vi "Manager Launcher.vi"() -> ()   [LabVIEW 2021, in "CIF Engine Launch.lvlib"]
uses:
  CIF Engine Launch.lvlib
  CIFUtilities/CIFLogs/Typedef/Message Type.ctl
  CIFUtilities/CIFConfigurationFile/typedef/Location Type.ctl
  363d3bde-6874-4068-849e-62e045d4c070.vi
  CIFUtilities/CIFConfigurationFile/CIF Configuration File Location.vi
  <vilib>/Comparison/Less/Less Functor/Less Functor.lvclass
  <vilib>/Utility/LVLibp/NI_PackedLibraryUtility.lvlib
  CIFUtilities/CIFConfigurationFile/CIF Configuration File.lvlib
  CIFUtilities/CIFLogs/CIFLogs.lvlib
panel:
  out "error out":errorcluster
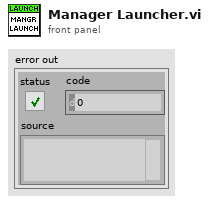
[diagram p1: front panel]
types:
  T1 = typedef "CIFLogs.lvlib/Message Type.ctl" = enum16{"Error", "Information", "Print Terminal", "Configuration"}
  T2 = enum32{"Invalid", "Standard", "Closed", "Hidden", "Minimized", "Maximized"}
  T3 = typedef "CIF Configuration File.lvlib/Location Type.ctl" = enum16{"Config File", "Manager", "Protos", "Plugins", "UI Plugins", "Logs", "Orchestrations"}
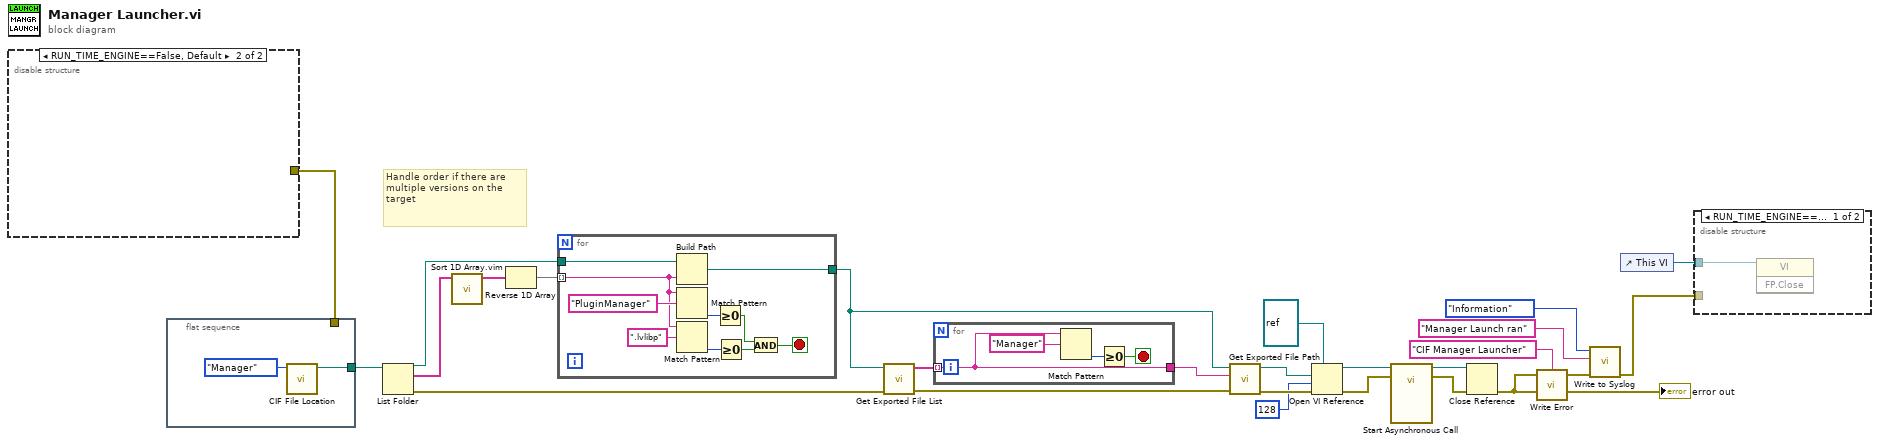
[diagram p0: block diagram]
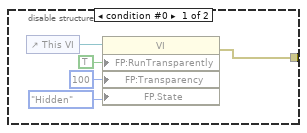
[diagram p2: hidden frame]
diagram:
  # "Handle order if there are multiple versions on the target"
  n1 = disable-structure shown="RUN_TIME_ENGINE==False, Default" {
    disable-tunnel: [w30 _] -> w9
    frame condition #0 {
      n2 = control-ref of="This VI"() -> (w31:refnum<vi>)
      n3 = property class="VI"(reference=w31, "FP:RunTransparently"=TRUE ("Front Panel Window:Run VI Transparently"), "FP:Transparency"=u8 100 ("Front Panel Window:Transparency"), "FP.State"=T2."Hidden" ("Front Panel Window:State")) -> (error out=w30:errorcluster)  [unwired: 1 in, 1 out]
    }
    frame condition #1 (active) {
    }
  }
  n4 = flat-sequence {
    tunnel: [w32] -> w10
    tunnel: w9 -> [_]
    frame #0 {
      n5 = call "CIF File Location.vi"("LocationType"=Location_Type."Manager") -> ("Location"=w32:path)  [unwired: 10 in]
    }
  }
  n6 = List Folder(path=w10) -> (path out=w25:path, filenames=w23:string[], error out=w26:errorcluster)  [unwired: 3 in, 1 out]
  n7 = call "Sort 1D Array.vim"("unsorted array"=w23) -> ("sorted array"=w22:string[])  [unwired: 10 in]
  n8 = Reverse 1D Array(array=w22) -> (reversed array=w21:string[])
  n9 = for {
    tunnel: w21 -> [w39] mode=indexing
    tunnel: [w40] -> w24
    tunnel: w25 -> [w41]
    stop <- w34 stop-if-true
    n10 = Build Path(base path=w41, name or relative path=w39) -> (appended path=w40:path)
    n11 = Match Pattern(string=w39, regular expression="PluginManager") -> (offset past match=w43:i32)  [unwired: 1 in, 3 out]
    n12 = Match Pattern(string=w39, regular expression=".lvlibp") -> (offset past match=w37:i32)  [unwired: 1 in, 3 out]
    n13 = Greater Or Equal To 0?(x=w43) -> (x >= 0?=w35:bool)
    n14 = Greater Or Equal To 0?(x=w37) -> (x >= 0?=w36:bool)
    n15 = And(x=w35, y=w36) -> (x .and. y?=w34:bool)
  }
  n16 = call <vilib>:"Get Exported File List.vi"("error in (no error)"=w26, "packed library path"=w24) -> ("error out"=w3:errorcluster, "qualified names"=w20:string[])  [unwired: 7 in, 1 out]
  n17 = for {
    tunnel: w20 -> [w44] mode=indexing
    tunnel: [w44] -> w12
    stop <- w46 stop-if-true
    n18 = Match Pattern(string=w44, regular expression="Manager") -> (offset past match=w47:i32)  [unwired: 1 in, 3 out]
    n19 = Greater Or Equal To 0?(x=w47) -> (x >= 0?=w46:bool)
  }
  n20 = call <vilib>:"Get Exported File Path.vi"("error in (no error)"=w3, "qualified name"=w12, "packed library path"=w24) -> ("error out"=w18:errorcluster, "path"=w19:path)  [unwired: 7 in]
  n21 = Open VI Reference(type specifier VI Refnum (for type only)=refnum<vi> refnum, vi path=w19, options=128, error in (no error)=w18) -> (vi reference=w16:refnum<vi>, error out=w15:errorcluster)  [unwired: 2 in]
  n22 = call-by-ref "Start Asynchronous Call"(reference=w16, error in=w15) -> (reference out=w14:refnum<vi>, error out=w13:errorcluster)  [unwired: 12 in]
  n23 = Close Reference(reference=w14, error in (no error)=w13) -> (error out=w1:errorcluster)
  "error out" <- w1
  n24 = call "Write Error.vi"("error in (no error)"=w1, "Plugin Name"="CIF Manager Launcher") -> ("cleared error"=w4:errorcluster)  [unwired: 2 in]
  n25 = call "Write to Syslog.vi"("error in (no error)"=w4, "message"="Manager Launch ran", "CIF Message Type"=Message_Type."Information") -> ("error out"=w7:errorcluster)  [unwired: 8 in]
  n26 = control-ref of="This VI"() -> (w11:refnum<vi>)
  n27 = disable-structure shown="RUN_TIME_ENGINE==True" {
    disable-tunnel: w11 -> [w48 _]
    disable-tunnel: w7 -> [_ _]
    frame condition #0 {
      n28 = invoke class="VI" method="FP.Close"(reference=w48) -> ()  [unwired: 2 in, 3 out]
    }
    frame condition #1 (active) {
    }
  }
